vi "Configure Record Parameters (5772).vi"(6 "Record Count":u16=1, 7 "Record Length":u16=3000, 8 "error in":errorcluster, 9 "% of Acquisition Hold Off Time":dbl=10.0, 10 "% of Pre-Trigger Samples":dbl=10.0, 11 "FPGA VI Reference In":refnum<k20>) -> (0 "error out":errorcluster, 3 "FPGA VI Reference Out":refnum<k20>, 4 "Actual Record Length":u16=3000)   [LabVIEW 2011]
uses:
  <vilib>/rvi/errors/niLvFpgaAdjustHostInterfaceError.vi
  <vilib>/rvi/interface/nirviReadWriteControl/nirviReadWriteControl.xnode
  NiFpgaLv.dll
  <vilib>/rvi/interface/Simulation/niFpgaSimulationCallBeginRW.vi
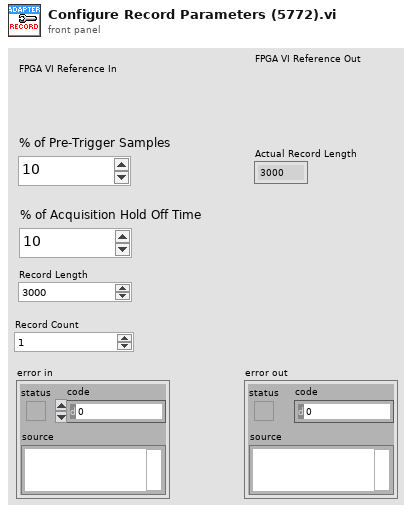
[diagram p1: front panel]
types:
  T1 = cluster{"Load Record Parameters?":bool, "Pre Trigger Samples":u16, "Samples per Record":u16, "Trigger Hold Off":u16, "Record Count":u16}
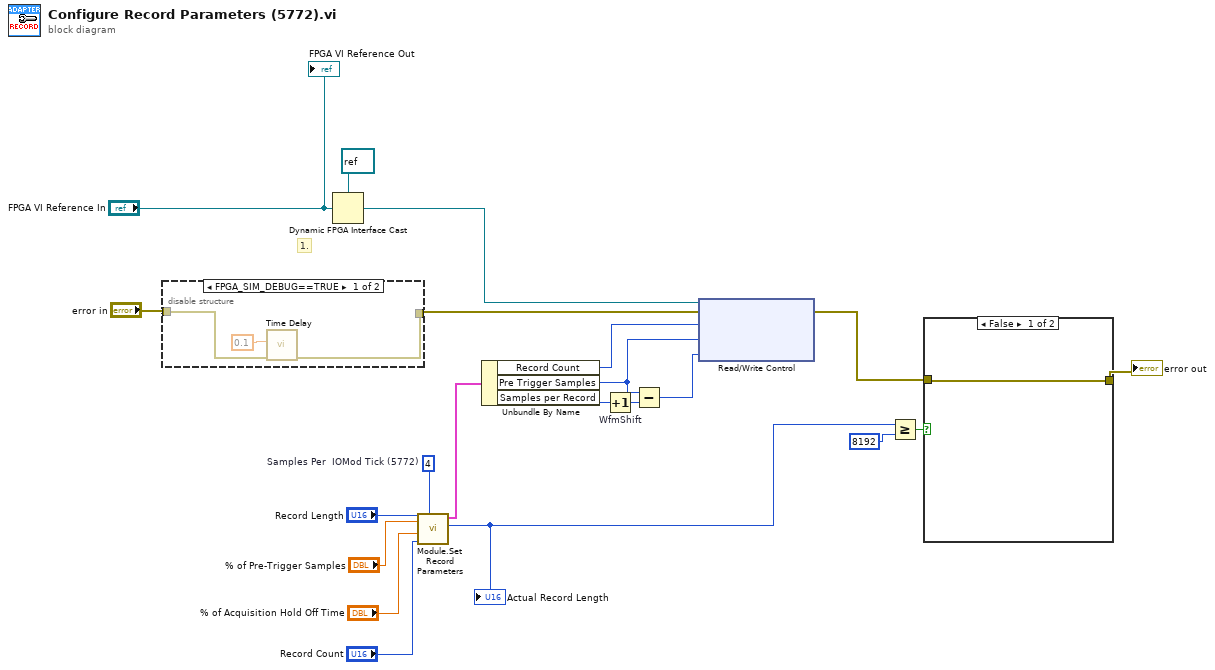
[diagram p0: block diagram]
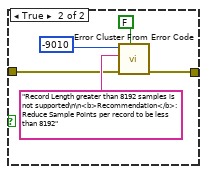
[diagram p3: hidden frame]
diagram:
  w2 = u16 4  # Samples Per  IOMod Tick (5772)
  # "1."
  n1 = disable-structure shown="FPGA_SIM_DEBUG==TRUE" {
    disable-tunnel: "error in" -> [w22 w25]
    disable-tunnel: [w23 w25] -> w10
    frame condition #0 {
      n2 = call "Time Delay"("error in (no error)"=w22, "Delay Time (s)"=0.1) -> ("error out"=w23:errorcluster)  [unwired: 9 in]
    }
    frame condition #1 (active) {
    }
  }
  n3 = Dynamic FPGA Interface Cast(Session In=refnum<k20> refnum ("Type"), Type="FPGA VI Reference In") -> (Session Out=w15:refnum<k20>)
  n4 = call <userlib>:"Module.Set Record Parameters.vi"("Samples Per  IOMod Tick"=w2, "Record Count"="Record Count", "% of Hold Off Time"="% of Acquisition Hold Off Time", "% of Pre-Trigger Samples"="% of Pre-Trigger Samples", "Total Number of Samples"="Record Length") -> ("Actual Record Length"=w8:u16, "Record Parameters"=w7:T1)  [unwired: 3 in, 2 out]
  "Actual Record Length" <- w8
  n5 = Unbundle By Name(w7) -> ("Record Count"=w6:u16, "Pre Trigger Samples"=w5:u16, "Samples per Record"=w4:u16)
  n6 = Increment "WfmShift"(x=w4) -> (x+1=w1:u16)
  n7 = Subtract(x=w5, y=w1) -> (x-y=w3:u16)
  n8 = xnode "Read/Write Control"("FPGA VI Reference In"=w15, "error in"=w10, "Record Count"=w6, "PreTrigger Samples"=w5, "PostTrigger Samples"=w3) -> ("error out"=w9:errorcluster)  [unwired: 1 out]
  n9 = Greater Or Equal?(x=w8, y=u16 8192) -> (x >= y?=w11:bool)
  n10 = case shown="False" w11 {
    tunnel: [w26 w31] -> w13
    tunnel: w9 -> [w26 w27]
    frame False {
    }
    frame True {
      n11 = call <vilib>:"Error Cluster From Error Code.vi"("show call chain? (False)"=FALSE, "error in (no error)"=w27, "error message (\"\")"="Record Length greater than 8192 samples is not supported\n\n<b>Recommendation</b>: Reduce Sample Points per record to be less than 8192" ("source"), "error code (0)"=-9010 ("code")) -> ("error out"=w31:errorcluster)  [unwired: 5 in]
    }
  }
  "error out" <- w13
  "FPGA VI Reference Out" <- "FPGA VI Reference In"
